vi "Initialize Attributes.vi"(8 "error in (no error)":errorcluster, 10 "Attribute Data":variant, 11 "CS++GoBangClient in":refnum<class "CS++GoBangClient.lvclass">) -> (0 "error out":errorcluster, 2 "Found?":bool, 3 "CS++GoBangClient out":refnum<class "CS++GoBangClient.lvclass">)   [LabVIEW 2014, in "GoBang.lvlib" / "CS++GoBangClient.lvclass"]
doc: "Initialize object attribute.\n\nUnique resources should be allocated elsewhere!"
uses:
  CS++GoBangClient.lvclass
  CSPP_Core/Classes/CS++ProcessVariables/SVConnection/SVConnection.lvclass
  CSPP_Core/Classes/CS++ProcessVariables/ProcessVariable/PV.lvclass
  CSPP_Core/Actors/CS++BaseActor/CS++BaseActor.lvclass/CS++BaseActor.ctl
  CSPP_Core/Classes/CS++ProcessVariables/ProcessVariable/PV.lvclass/PV.ctl
  CSPP_Core/Classes/CS++ProcessVariables/PVConnection/PVConnection.lvclass/PVConnection.ctl
  CS++GoBangClient.lvclass/CS++GoBangClient.ctl
  CSPP_Core/Actors/CS++BaseActor/CS++BaseActor.lvclass
  CSPP_Core/Classes/CS++BaseClasses/Factory/CS++Factory.lvclass
  CSPP_Core/Classes/CS++ProcessVariables/PVConnection/PVConnection.lvclass
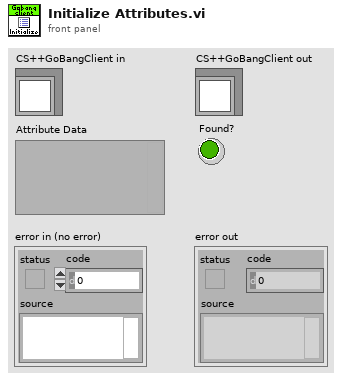
[diagram p1: front panel]
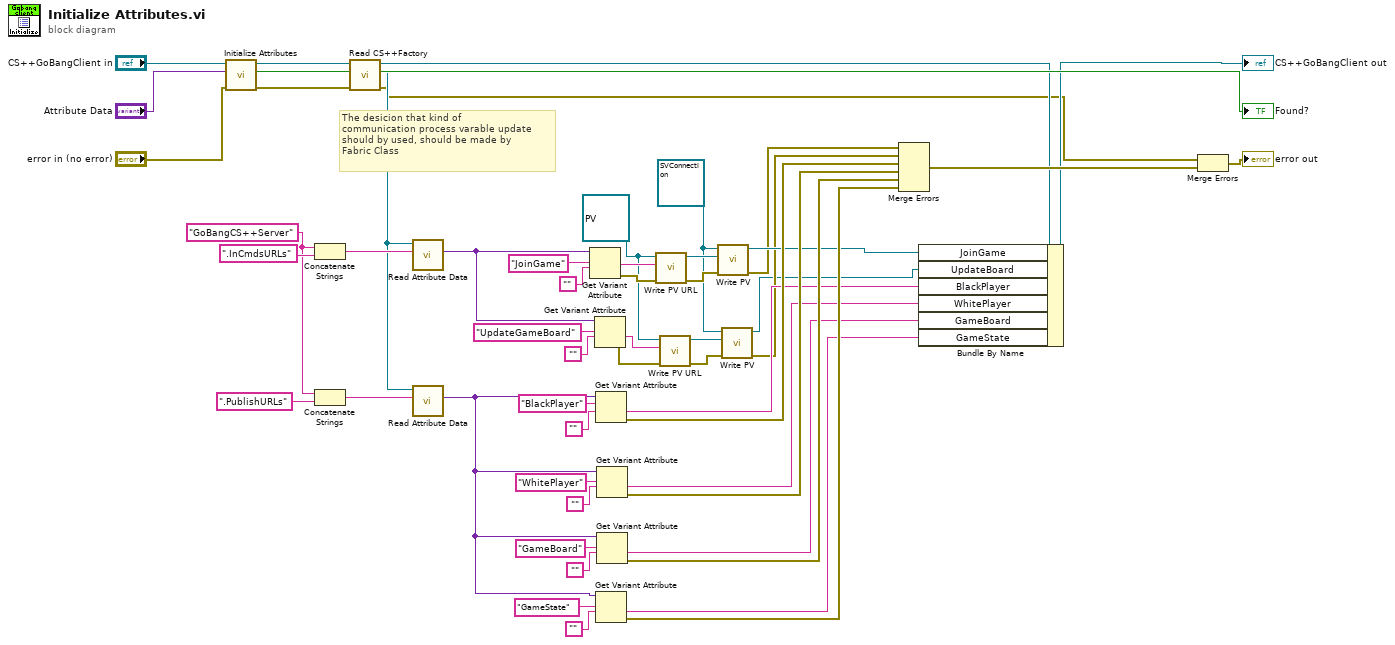
[diagram p0: block diagram]
diagram:
  w4 = refnum<class "PV.lvclass"> refnum ("CS++ProcessVariables.lvlib:PV.lvclass")
  w33 = "GoBangCS++Server" ("string")
  w3 = refnum<class "SVConnection.lvclass"> refnum ("CS++ProcessVariables.lvlib:SVConnection.lvclass")
  # "The desicion that kind of\ncommunication process varable update \nshould by used, should be made by \nFabric Class"
  n1 = call-parent "Initialize Attributes.vi"("error in (no error)"="error in (no error)", "Attribute Data"="Attribute Data", "CS++BaseActor in"="CS++GoBangClient in") -> ("error out"=w16:errorcluster, "Found?"=→"Found?":bool, "CS++BaseActor out"=w19:refnum<class "CS++GoBangClient.lvclass">)  [unwired: 6 in]
  n2 = Concatenate Strings(w33, ".InCmdsURLs" ("string")) -> (w50:string)
  n3 = Concatenate Strings(w33, ".PublishURLs" ("string")) -> (w39:string)
  n4 = call "Read CS++Factory.vi"("error in (no error)"=w16, "CS++BaseActor in"=w19) -> ("error out"=w15:errorcluster, "CS++Factory"=w36:refnum<class "CS++Factory.lvclass">, "CS++BaseActor out"=w30:refnum<class "CS++GoBangClient.lvclass">)  [unwired: 7 in]
  n5 = call-dynamic "Read Attribute Data.vi"("Object Name"=w50, "CS++Factory in"=w36) -> ("Attribute Data"=w40:variant)  [unwired: 7 in, 2 out]
  n6 = call-dynamic "Read Attribute Data.vi"("Object Name"=w39, "CS++Factory in"=w36) -> ("Attribute Data"=w26:variant)  [unwired: 7 in, 2 out]
  n7 = Get Variant Attribute(Variant=w40, name="JoinGame", default value (empty Variant)="") -> (value=w9:string, error out=w12:errorcluster)  [unwired: 1 in, 2 out]
  n8 = Get Variant Attribute(Variant=w40, name="UpdateGameBoard", default value (empty Variant)="") -> (value=w2:string, error out=w1:errorcluster)  [unwired: 1 in, 2 out]
  n9 = Get Variant Attribute(Variant=w26, name="BlackPlayer", default value (empty Variant)="") -> (value=w24:string, error out=w45:errorcluster)  [unwired: 1 in, 2 out]
  n10 = Get Variant Attribute(Variant=w26, name="GameState", default value (empty Variant)="") -> (value=w21:string, error out=w25:errorcluster)  [unwired: 1 in, 2 out]
  n11 = Get Variant Attribute(Variant=w26, name="WhitePlayer", default value (empty Variant)="") -> (value=w23:string, error out=w41:errorcluster)  [unwired: 1 in, 2 out]
  n12 = Get Variant Attribute(Variant=w26, name="GameBoard", default value (empty Variant)="") -> (value=w22:string, error out=w34:errorcluster)  [unwired: 1 in, 2 out]
  n13 = call "Write PV URL.vi"("error in (no error)"=w12, "PV URL"=w9, "PV in"=w4) -> ("error out"=w13:errorcluster, "PV out"=w14:refnum<class "PV.lvclass">)  [unwired: 7 in]
  n14 = call "Write PV URL.vi"("error in (no error)"=w1, "PV URL"=w2, "PV in"=w4) -> ("error out"=w8:errorcluster, "PV out"=w7:refnum<class "PV.lvclass">)  [unwired: 7 in]
  n15 = call "Write PV.vi"("error in (no error)"=w13, "PV"=w14, "PVConnection in"=w3) -> ("error out"=w10:errorcluster, "PVConnection out"=w11:refnum<class "SVConnection.lvclass">)  [unwired: 7 in]
  n16 = call "Write PV.vi"("error in (no error)"=w8, "PV"=w7, "PVConnection in"=w3) -> ("error out"=w6:errorcluster, "PVConnection out"=w5:refnum<class "SVConnection.lvclass">)  [unwired: 7 in]
  n17 = Merge Errors(w10, w6, w45, w41, w34, w25) -> (w31:errorcluster)
  n18 = Bundle By Name(cluster=w30, "JoinGame"=w11, "UpdateBoard"=w5, "BlackPlayer"=w24, "WhitePlayer"=w23, "GameBoard"=w22, "GameState"=w21) -> (→"CS++GoBangClient out":refnum<class "CS++GoBangClient.lvclass">)
  n19 = Merge Errors(w15, w31) -> (→"error out":errorcluster)
